vi "Acquire.vi"(6 "Acquisition":refnum<queue>, 7 "Longueur d'onde":dbl, 8 "error in (no error)":errorcluster, 9 "Data Queue":refnum<queue>, 10 "Data Notifier":refnum<notifier>) -> (0 "error out":errorcluster, 3 "Disconnected":bool=TRUE)   [LabVIEW 2018, in "Acquisition.lvlib"]
doc: "Perform the acquisition. Replace the contents of this diagram with calls to acquisition hardware."
uses:
  Acquisition.lvlib
  support/Message Queue/Message Cluster.ctl
  support/Message Queue/Message Queue.lvlib
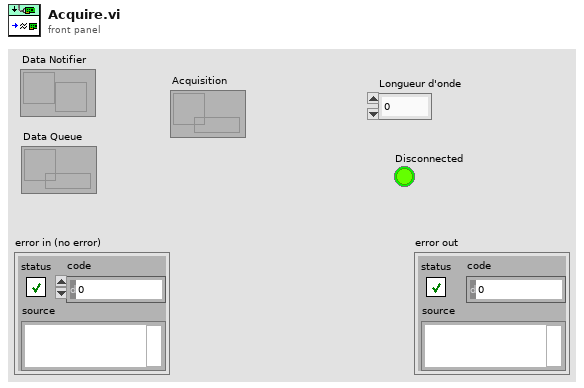
[diagram p1: front panel]
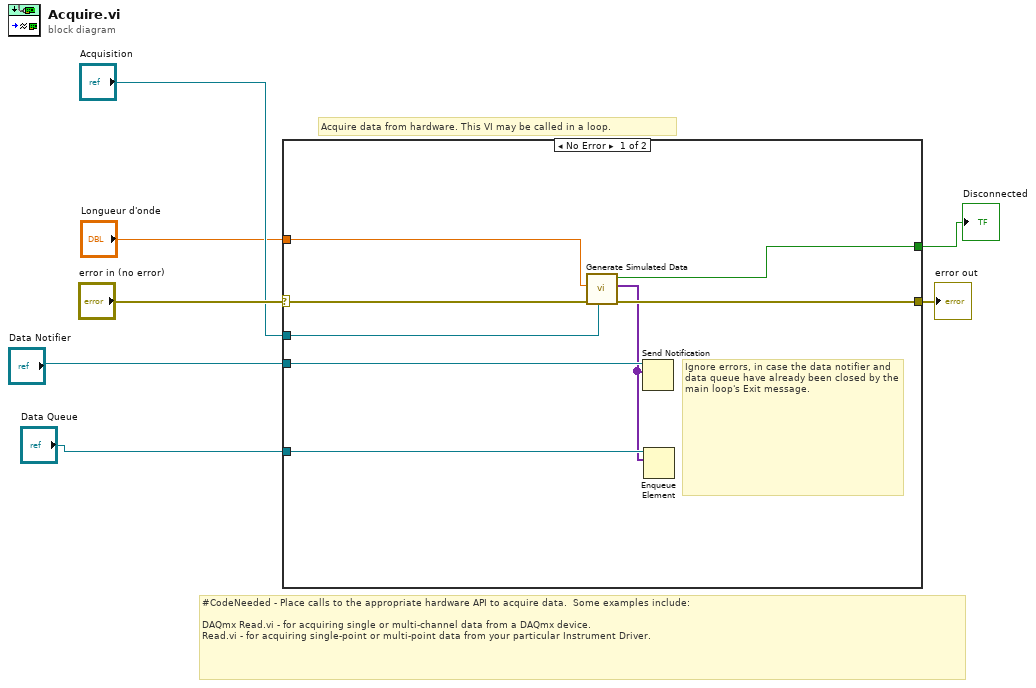
[diagram p0: block diagram]
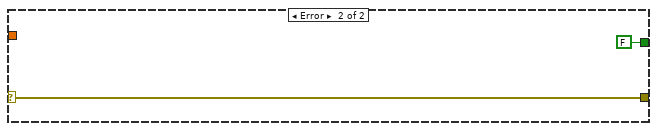
[diagram p2: hidden frame]
diagram:
  # "Acquire data from hardware. This VI may be called in a loop."
  # "#CodeNeeded - Place calls to the appropriate hardware API to acquire data.  Some examples include:\n\nDAQmx Read.vi - for acquiring single or multi-channel data from a DAQmx device.\nRead.vi - for acquiring single-point or multi-point data from your particular Instrument Driver."
  n1 = case shown="No Error" "error in (no error)" {
    selector: "error in (no error)" -> [w15 w17]
    tunnel: [w12 w17] -> w6
    tunnel: "Data Notifier" -> [w14 _]
    tunnel: "Data Queue" -> [w13 _]
    tunnel: "Acquisition" -> [w11 _]
    tunnel: "Longueur d'onde" -> [w10 _]
    tunnel: [w8 FALSE ("Disconnected")] -> w1
    frame No Error {
      # "Ignore errors, in case the data notifier and data queue have already been closed by the main loop's Exit message."
      n2 = call "Generate Simulated Data.vi"("Acquisition"=w11, "error in (no error)"=w15, "Longueur d'onde"=w10) -> ("error out"=w12:errorcluster, "Data Out"=w9:variant[], "Disconnected"=w8:bool)  [unwired: 6 in]
      n3 = Send Notification(notification=w9, notifier=w14) -> ()  [unwired: 1 in, 2 out]
      n4 = Enqueue Element(queue=w13, element=w9) -> ()  [unwired: 2 in, 3 out]
    }
    frame Error {
    }
  }
  "error out" <- w6
  "Disconnected" <- w1
